vi "AutonomousDist.vi"(10 "Distance":dbl format="%#_13g", 11 "Speed":dbl format="%#_13g") -> ()   [LabVIEW 2014]
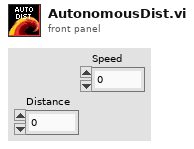
[diagram p1: front panel]
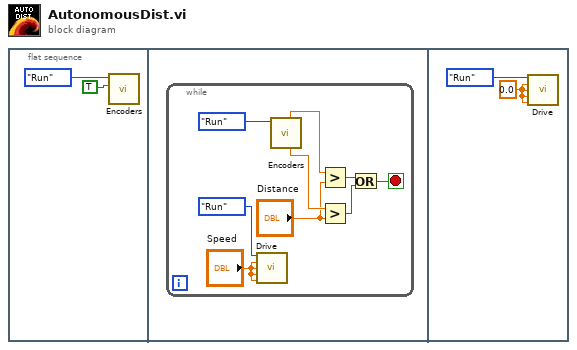
[diagram p0: block diagram]
diagram:
  n1 = flat-sequence {
    frame #0 {
      n2 = call "Encoders.vi"("Reset"=TRUE, "Enum"=enum16{"Start", "Run", "End"}."Run") -> ()  [unwired: 4 in, 6 out]
    }
    frame #1 {
      n3 = while {
        stop <- w5 stop-if-true
        n4 = call "Drive.vi"("Enum"=enum16{"Start", "Run", "End"}."Run", "Left Primary"="Speed", "Left Secondary"="Speed", "Right Primary"="Speed", "Right Secondary"="Speed") -> ()  [unwired: 11 in]
        n5 = call "Encoders.vi"("Enum"=enum16{"Start", "Run", "End"}."Run") -> ("LDistance"=w8:dbl, "RDistance"=w9:dbl)  [unwired: 5 in, 4 out]
        n6 = Greater?(x=w9, y="Distance") -> (0:w7:bool)
        n7 = Greater?(x=w8, y="Distance") -> (0:w6:bool)
        n8 = Or(x=w7, y=w6) -> (x .or. y?=w5:bool)
      }
    }
    frame #2 {
      w12 = 0.0
      n9 = call "Drive.vi"("Enum"=enum16{"Start", "Run", "End"}."Run", "Left Primary"=w12, "Left Secondary"=w12, "Right Primary"=w12, "Right Secondary"=w12) -> ()  [unwired: 11 in]
    }
  }
